vi "Steppers_simultaneous_v2.vi"() -> ()   [LabVIEW 2019]
uses:
  <vilib>/Instr/_visa.llb/VISA Set IO Buffer Mask.ctl
  <vilib>/Instr/_visa.llb/VISA Configure Serial Port (Instr).vi
panel:
  in  "Light 1":i32 min=0 max=1 format="%01.0f"
  out "resulting string":string
  in  "Light 2":i32 min=0 max=1 format="%01.0f"
  in  "Light 3":i32 min=0 max=1 format="%01.0f"
  in  "Fans":i32 min=0 max=1 format="%01.0f"
  in  "Motor 10":i32 min=0 max=99999 format="%05.0f"
  in  "Motor 9":i32 min=0 max=99999 format="%05.0f"
  in  "Motor 8":i32 min=0 max=99999 format="%05.0f"
  in  "Motor 7":i32 min=0 max=99999 format="%05.0f"
  in  "Motor 6":i32 min=0 max=99999 format="%05.0f"
  in  "Motor 5":i32 min=0 max=99999 format="%05.0f"
  in  "Motor 4":i32 min=0 max=99999 format="%05.0f"
  in  "Motor 3":i32 min=0 max=99999 format="%05.0f"
  in  "Motor 2":i32 min=0 max=99999 format="%05.0f"
  in  "Motor 1":i32 min=0 max=99999 format="%05.0f"
  in  "VISA resource name":refnum<visa-resource-name>
  in  "stop":bool
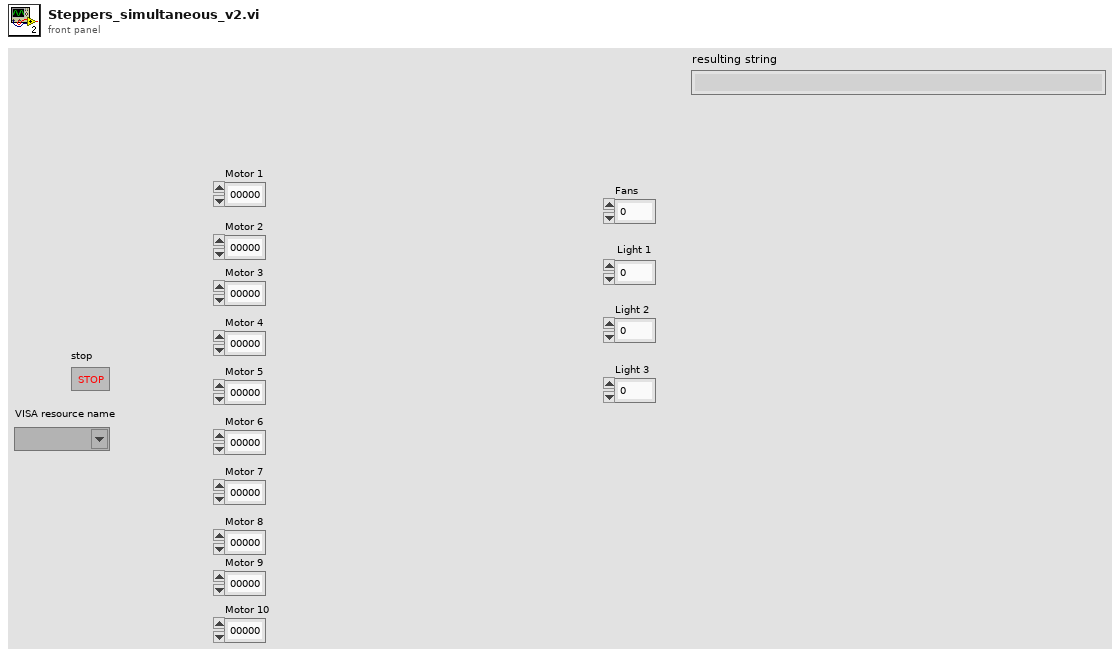
[diagram p1: front panel]
types:
  T1 = typedef "VISA Set IO Buffer Mask.ctl" = u16
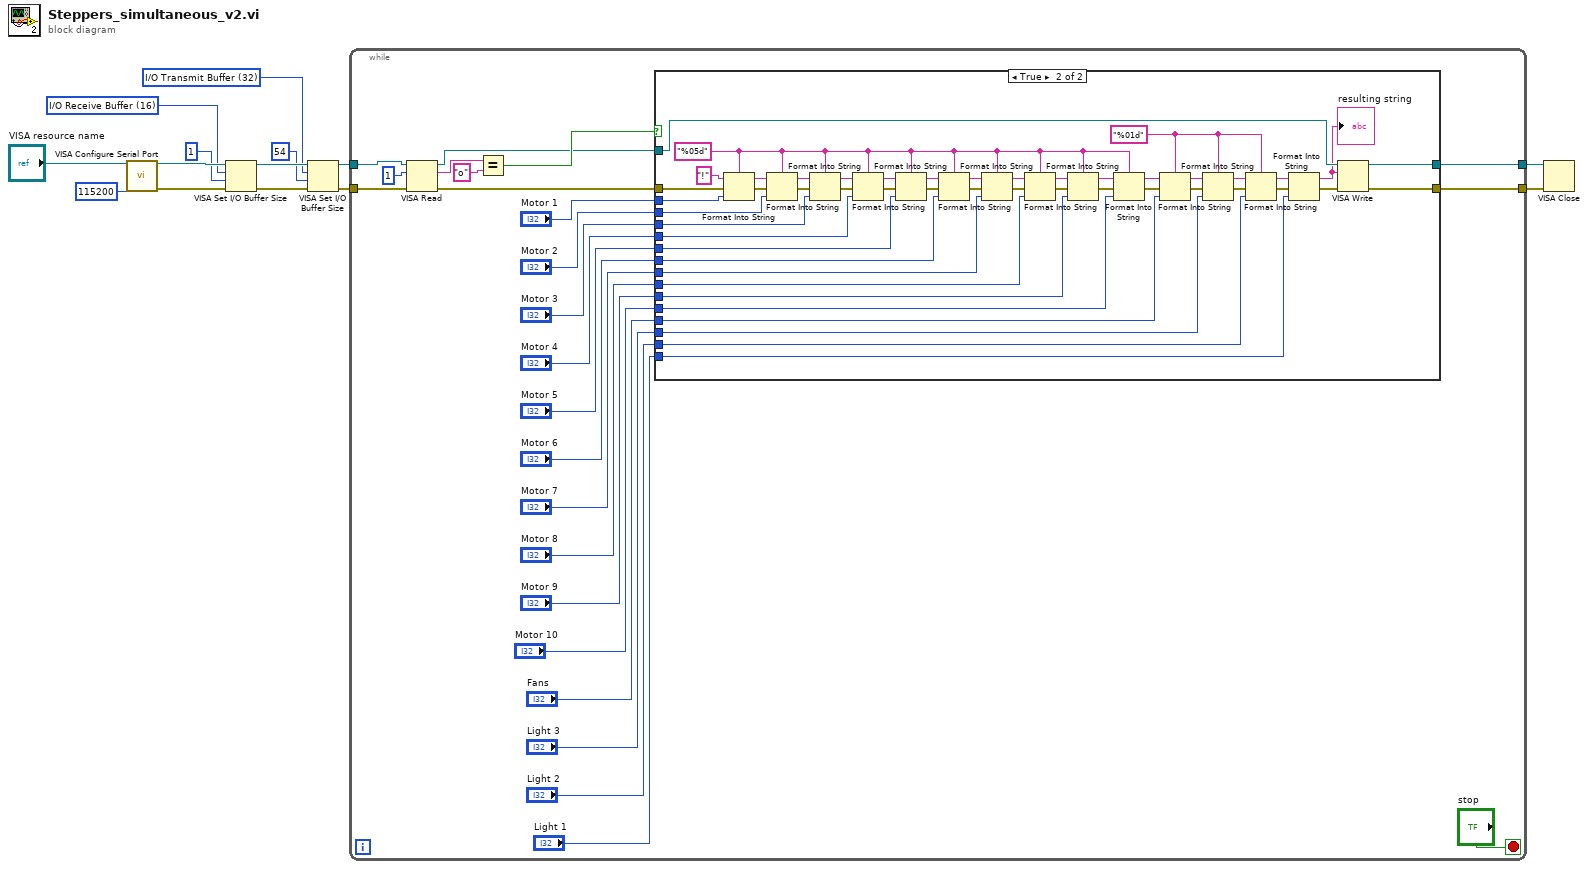
[diagram p0: block diagram]
diagram:
  w3 = T1 32 items=["I/O Receive Buffer"=16, "I/O Transmit Buffer"=32, "I/O Receive and Transmit Buffer"=48] ("Mask")
  w8 = T1 16 items=["I/O Receive Buffer"=16, "I/O Transmit Buffer"=32, "I/O Receive and Transmit Buffer"=48] ("Mask")
  n1 = call-poly "VISA Configure Serial Port"("VISA resource name"="VISA resource name", "baud rate (9600)"=u32 115200) -> ("VISA resource name out"=w11:refnum<visa-resource-name>, "error out"=w10:errorcluster)  [unwired: 12 in]
  n2 = VISA Set I/O Buffer Size(VISA resource name=w11, mask (16)=w8, size (4096)=u32 1, error in (no error)=w10) -> (VISA resource name out=w6:refnum<visa-resource-name>, error out=w7:errorcluster)
  n3 = VISA Set I/O Buffer Size(VISA resource name=w6, mask (16)=w3, size (4096)=u32 54, error in (no error)=w7) -> (VISA resource name out=w5:refnum<visa-resource-name>, error out=w4:errorcluster)
  n4 = while {
    tunnel: w4 -> [w30]
    tunnel: w5 -> [w29]
    tunnel: [w31] -> w13
    tunnel: [w32] -> w12
    stop <- "stop" stop-if-true
    n5 = VISA Read(VISA resource name=w29, byte count=u32 1, error in (no error)=w30) -> (VISA resource name out=w35:refnum<visa-resource-name>, read buffer=w34:string, error out=w36:errorcluster)  [unwired: 1 out]
    n6 = Equal?(x=w34, y="o") -> (x = y?=w37:bool)
    n7 = case shown="True" w37 {
      tunnel: w35 -> [w40 w75]
      tunnel: w36 -> [w41 w72]
      tunnel: [w40 w74] -> w32
      tunnel: [w41 w73] -> w31
      tunnel: "Motor 1" -> [_ w71]
      tunnel: "Motor 2" -> [_ w70]
      tunnel: "Motor 3" -> [_ w69]
      tunnel: "Motor 4" -> [_ w68]
      tunnel: "Motor 5" -> [_ w67]
      tunnel: "Motor 6" -> [_ w66]
      tunnel: "Motor 7" -> [_ w65]
      tunnel: "Motor 8" -> [_ w64]
      tunnel: "Motor 9" -> [_ w63]
      tunnel: "Motor 10" -> [_ w62]
      tunnel: "Fans" -> [_ w56]
      tunnel: "Light 2" -> [_ w55]
      tunnel: "Light 3" -> [_ w54]
      tunnel: "Light 1" -> [_ w46]
      frame False {
      }
      frame True {
        w47 = "%01d" ("format string")
        w57 = "%05d" ("format string")
        n8 = Format Into String(format string=w57, initial string="!" ("write buffer"), error in=w72, w71) -> (resulting string=w89:string, error out=w90:errorcluster)
        n9 = Format Into String(format string=w57, initial string=w89, error in=w90, w70) -> (resulting string=w87:string, error out=w88:errorcluster)
        n10 = Format Into String(format string=w57, initial string=w87, error in=w88, w69) -> (resulting string=w85:string, error out=w86:errorcluster)
        n11 = Format Into String(format string=w57, initial string=w85, error in=w86, w68) -> (resulting string=w83:string, error out=w84:errorcluster)
        n12 = Format Into String(format string=w57, initial string=w83, error in=w84, w67) -> (resulting string=w81:string, error out=w82:errorcluster)
        n13 = Format Into String(format string=w57, initial string=w81, error in=w82, w66) -> (resulting string=w79:string, error out=w80:errorcluster)
        n14 = Format Into String(format string=w57, initial string=w79, error in=w80, w65) -> (resulting string=w78:string, error out=w77:errorcluster)
        n15 = Format Into String(format string=w57, initial string=w78, error in=w77, w64) -> (resulting string=w59:string, error out=w61:errorcluster)
        n16 = Format Into String(format string=w57, initial string=w59, error in=w61, w63) -> (resulting string=w58:string, error out=w60:errorcluster)
        n17 = Format Into String(format string=w57, initial string=w58, error in=w60, w62) -> (resulting string=w50:string, error out=w53:errorcluster)
        n18 = Format Into String(format string=w47, initial string=w50, error in=w53, w56) -> (resulting string=w49:string, error out=w52:errorcluster)
        n19 = Format Into String(format string=w47, initial string=w49, error in=w52, w54) -> (resulting string=w48:string, error out=w51:errorcluster)
        n20 = Format Into String(format string=w47, initial string=w48, error in=w51, w55) -> (resulting string=w44:string, error out=w45:errorcluster)
        n21 = Format Into String(initial string=w44, error in=w45, w46) -> (resulting string=w42:string, error out=w43:errorcluster)  [unwired: 1 in]
        "resulting string" <- w42
        n22 = VISA Write(VISA resource name=w75, write buffer=w42, error in (no error)=w43) -> (VISA resource name out=w74:refnum<visa-resource-name>, error out=w73:errorcluster)  [unwired: 1 out]
      }
    }
  }
  n23 = VISA Close(VISA resource name=w12, error in (no error)=w13) -> ()  [unwired: 1 out]
